vi "Example Kafka Read Events Data - Real Time.vi"() -> ()   [LabVIEW 2019]
doc: "This example demonstrates how to read measured data, text and timestamps from a .tdms file using the TDMS API."
uses:
  support/_readType.ctl
panel:
  out "Exit":bool
  in  "Stop":bool
  out "Property Values":variant[][](array[variant])
  out "Property Names":string[][](array[string])
  out "Measured Data":waveform(dbl)[](graph)
  # "Overview: Demonstrates the use of the TDMS Read function to read measured data, text and timestamps from an existing .tdms file.\nInstructions:\n1. Make sure you have already run TDMS Write Events Data.vi.\n2. Run this VI.\n3. Delete the .tdms file (located at [LabVIEW Data]\\Example Events Data.tdms) when you are done."
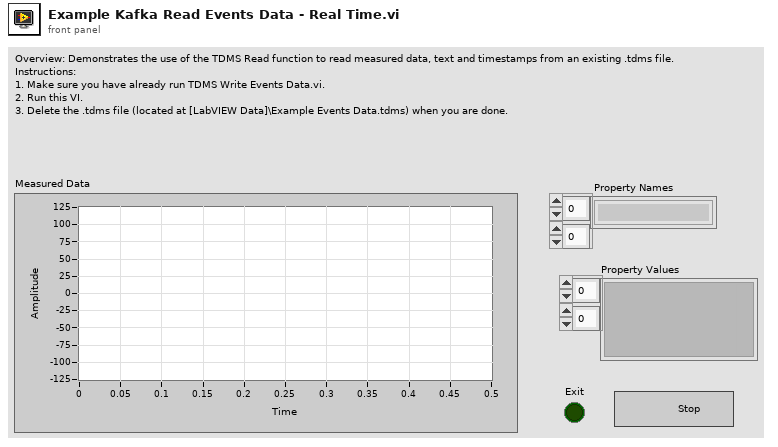
[diagram p1: front panel]
types:
  T1 = typedef "_readType.ctl" = enum16{"All", "Real-time", "Start Offset"}
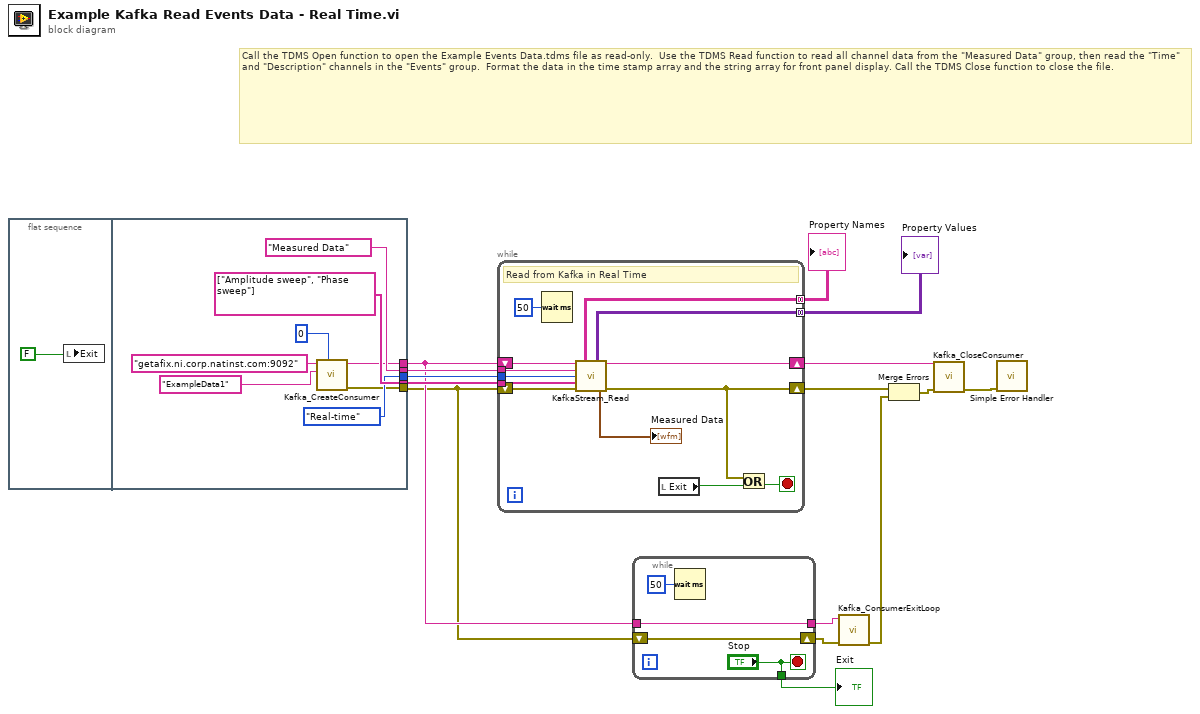
[diagram p0: block diagram]
diagram:
  # "Call the TDMS Open function to open the Example Events Data.tdms file as read-only.  Use the TDMS Read function to read all channel data from the \"Measured Data\" group, then read the \"Time\" and \"Description\" channels in the \"Events\" group.  Format the data in the time stamp array and the string array for front panel display. Call the TDMS Close function to close the file."
  n1 = flat-sequence {
    tunnel: ["Measured Data" ("group name")] -> w15
    tunnel: [string[] ["Amplitude sweep", "Phase sweep"] ("channel names")] -> w14
    tunnel: [_readType."Real-time" ("Read Type")] -> w11
    tunnel: [w18] -> w8
    tunnel: [w17] -> w6
    frame #0 {
      n2 = local write "Exit"(FALSE) -> ()
    }
    frame #1 {
      n3 = call "Kafka_CreateConsumer.vi"("Partition"=0, "Topic"="ExampleData1", "Kafka Broker"="getafix.ni.corp.natinst.com:9092") -> ("error out"=w17:errorcluster, "Consumer Handle"=w18:string)  [unwired: 7 in]
    }
  }
  n4 = while {
    tunnel: w15 -> [w35]
    tunnel: w14 -> [w34]
    tunnel: w11 -> [w31]
    tunnel: [w30] -> w10 mode=concatenating
    tunnel: [w29] -> w9 mode=concatenating
    shift-right: [w27] -> w4
    shift-left: w6 -> [w37]
    shift-right: [w32] -> w13
    shift-left: w8 -> [w36]
    stop <- w26 stop-if-true
    # "Read from Kafka in Real Time"
    n5 = Wait (ms)(milliseconds to wait=u32 50) -> ()  [unwired: 1 out]
    n6 = call "KafkaStream_Read.vi"("Consumer Handle"=w36, "Group Name"=w35, "Read Type"=w31, "Channel Names"=w34, "error in (no error)"=w37) -> ("Property Names"=w30:string[][], "Property Values"=w29:variant[][], "Consumer Handle Out"=w32:string, "Waveforms"=→"Measured Data":waveform(dbl)[], "error out"=w27:errorcluster)  [unwired: 4 in, 2 out]
    n7 = local read "Exit"() -> (w25:bool)
    n8 = Or(x=w27, y=w25) -> (x .or. y?=w26:bool)
  }
  "Property Names" <- w10
  "Property Values" <- w9
  n9 = while {
    tunnel: w8 -> [w40]
    tunnel: [w40] -> w7
    shift-right: [w39] -> w5
    shift-left: w6 -> [w39]
    tunnel: ["Stop"] -> w1
    stop <- "Stop" stop-if-true
    n10 = Wait (ms)(milliseconds to wait=u32 50) -> ()  [unwired: 1 out]
  }
  "Exit" <- w1
  n11 = call "Kafka_ConsumerExitLoop.vi"("error in (no error)"=w5, "Consumer Handle"=w7) -> ("error out"=w3:errorcluster)  [unwired: 8 in, 1 out]
  n12 = Merge Errors(w4, w3) -> (w2:errorcluster)
  n13 = call "Kafka_CloseConsumer.vi"("error in (no error)"=w2, "Consumer Handle"=w13) -> ("error out"=w12:errorcluster)  [unwired: 8 in, 1 out]
  n14 = call <vilib>:"Simple Error Handler.vi"("error in (no error)"=w12) -> ()  [unwired: 2 in, 7 out]
